vi "YARIC.vi"() -> ()   [LabVIEW 2014]
uses:
  <vilib>/Utility/file.llb/Read From Spreadsheet File (DBL).vi
  <vilib>/Waveform/WDTOps.llb/WDT Get Waveform Subset DBL.vi
  <vilib>/Utility/file.llb/Write To Spreadsheet File (DBL).vi
panel:
  in  "Right":dbl format="%#_13e"
  in  "Left":dbl format="%#_13e"
  # "Yet\nAnother\nRange\nInteger\nCalculator"
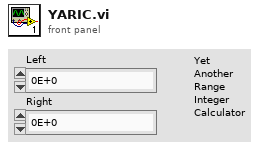
[diagram p1: front panel]
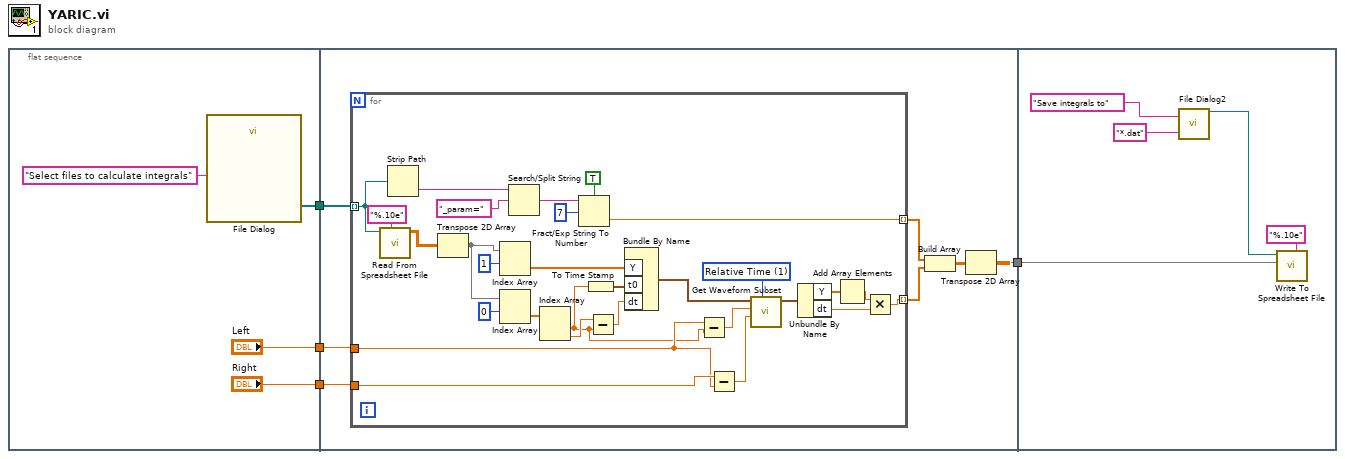
[diagram p0: block diagram]
diagram:
  n1 = flat-sequence {
    tunnel: [w8] -> w4
    tunnel: ["Left"] -> w3
    tunnel: ["Right"] -> w2
    tunnel: w4 -> [w13]
    tunnel: w3 -> [w15]
    tunnel: w2 -> [w14]
    tunnel: [w9] -> w1
    tunnel: w1 -> [w45]
    frame #0 {
      n2 = call "File Dialog"("prompt"="Select files to calculate integrals") -> ("selected paths"=w8:path[])  [unwired: 11 in, 3 out]
    }
    frame #1 {
      n3 = for {
        tunnel: w13 -> [w38] mode=indexing
        tunnel: [w22] -> w11 mode=indexing
        tunnel: w15 -> [w18]
        tunnel: w14 -> [w40]
        tunnel: [w32] -> w10 mode=indexing
        w44 = u16 1 items=["Samples", "Relative Time"] ("start/duration format")
        n4 = call-poly <vilib>:"Read From Spreadsheet File.vi"("format (%.3f)"="%.10e", "file path (dialog if empty)"=w38) -> ("all rows"=w31:dbl[][])  [unwired: 5 in, 4 out]
        n5 = Strip Path(path=w38) -> (name=w33:string)  [unwired: 1 out]
        n6 = Transpose 2D Array(2D array=w31) -> (transposed array=w28:dbl[][])
        n7 = Index Array(array=w28, index (row)=1) -> (element=w29:dbl[])  [unwired: 1 in]
        n8 = Index Array(array=w28, index (row)=0) -> (element=w26:dbl[])  [unwired: 1 in]
        n9 = Search/Split String(string=w33, search string/char (-)="_param=") -> (match + rest of string=w37:string)  [unwired: 1 in, 2 out]
        n10 = Index Array(array=w26) -> (element #1=w17:dbl, element #2=w23:dbl)  [unwired: 2 in]
        n11 = Fract/Exp String To Number(use system decimal point (T)=TRUE, string=w37, offset=7 ("offset (0)")) -> (number=w32:dbl)  [unwired: 1 in, 1 out]
        n12 = To Time Stamp(1:w17) -> (0:w25:timestamp)
        n13 = Subtract(x=w23, y=w17) -> (x-y=w24:dbl)
        n14 = Bundle By Name("Y"=w29, "t0"=w25, "dt"=w24) -> (w39:waveform(dbl))  [unwired: 1 in]
        n15 = Subtract(x=w18, y=w17) -> (x-y=w19:dbl)
        n16 = Subtract(x=w40, y=w18) -> (x-y=w41:dbl)
        n17 = call-poly <vilib>:"Get Waveform Subset.vi"("start/duration format"=w44, "duration"=w41, "start samples/time"=w19, "waveform in"=w39) -> ("waveform out"=w42:waveform(dbl))  [unwired: 2 in, 3 out]
        n18 = Unbundle By Name(w42) -> ("Y"=w43:dbl[], "dt"=w20:dbl)
        n19 = Add Array Elements(numeric array=w43) -> (sum=w21:dbl)
        n20 = Multiply(x=w21, y=w20) -> (x*y=w22:dbl)
      }
      n21 = Build Array(w10, w11) -> (w12:dbl[][])
      n22 = Transpose 2D Array(2D array=w12) -> (transposed array=w9:dbl[][])
    }
    frame #2 {
      n23 = call "File Dialog2"("prompt"="Save integrals to", "pattern (all files)"="*.dat") -> ("selected path"=w46:path)  [unwired: 10 in, 3 out]
      n24 = call-poly <vilib>:"Write To Spreadsheet File.vi"("format (%.3f)"="%.10e", "2D data"=w45, "file path (dialog if empty)"=w46) -> ()  [unwired: 5 in, 1 out]
    }
  }
